vi "GetShpaeResultValue.vi"(8 "error in (no error)":errorcluster, 10 "data":variant, 11 "SetParameter":T1={"Enum_ShapeType"=enum."Circles", "MaxParticle"=1, "Descriptor"={"Set 1"=100.0, "Set 2"=10.0, "Set 3"=200.0, "Set 4"=10.0}, "Match Options"={"Rotation"=TRUE, "Scale"=FALSE, "Occlusion"=FALSE, "Range Settings"=[{"Match Constraints"=0, "Min"=0.0, "Max"=360.0}]}, "Curve Parameters"={"Extraction Mode"=0, "Edge Threshold"=75, "Edge Filter Size"=1, "Min Length"=25, "Row Search Step Size"=15, "Col Search Step Size"=15, "Max Endpoint Gap"=10, "Closed"=FALSE, "Subpixel"=FALSE}, " score"=500.0} {"score" format="%#_15g"; "Curve Parameters"."Extraction Mode" items=["Normal", "Uniform Regions"]; "Curve Parameters"."Edge Filter Size" items=["Fine", "Normal"]; "Match Options"."Range Settings"."Match Constraints" items=["Rotation Angle (degrees)", "Scale Factor (%)", "Occlusion (%)"]}) -> (0 "error out":errorcluster, 3 "ResultValues":string[](array[string]))   [LabVIEW 2019]
uses:
  Controls/ShapeDectect/Analysis_ShapeDectect_Parameter.ctl
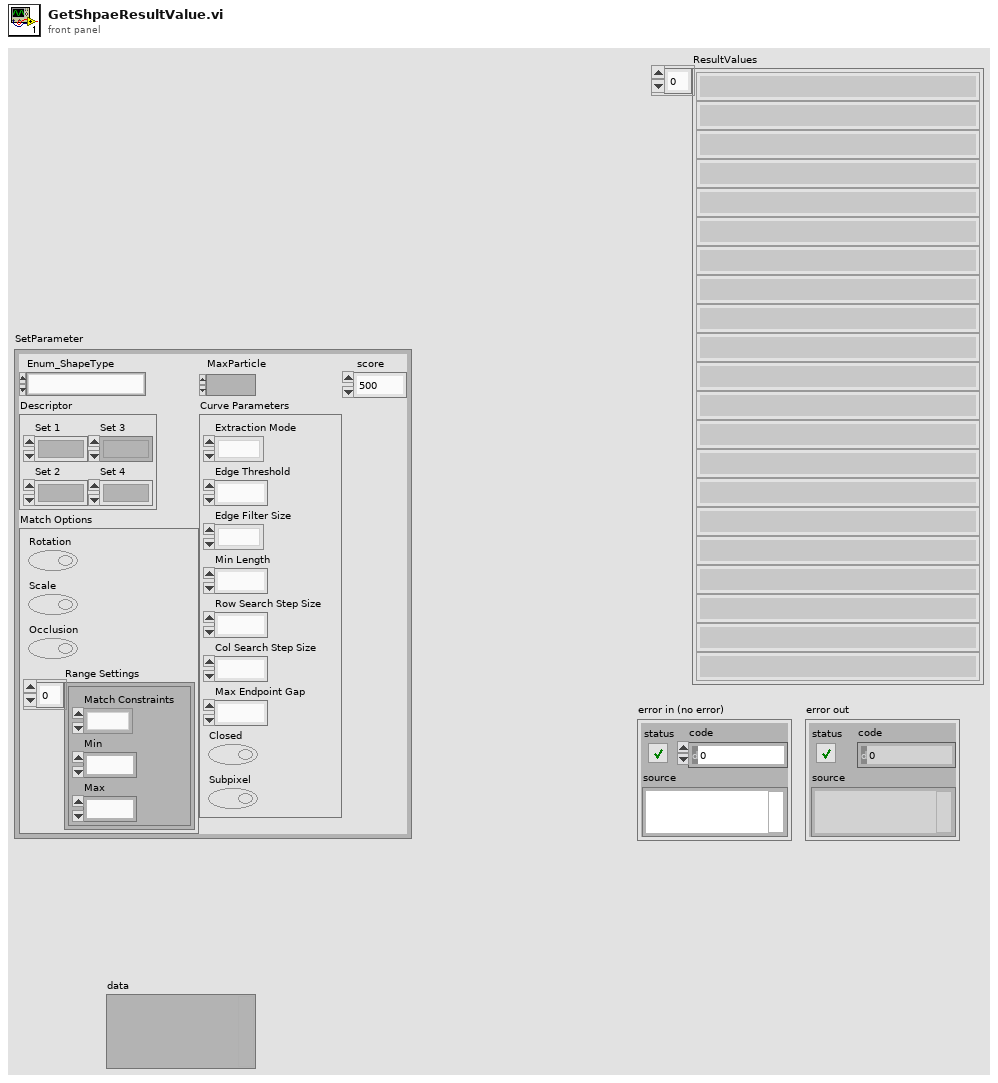
[diagram p1: front panel]
types:
  T1 = typedef "Analysis_ShapeDectect_Parameter.ctl" = cluster{"Enum_ShapeType":enum16{"Circles", "Ellipses", "Lines", "Rectangles"}, "MaxParticle":i32, "Descriptor":cluster{"Set 1":dbl, "Set 2":dbl, "Set 3":dbl, "Set 4":dbl}, "Match Options":cluster{"Rotation":bool, "Scale":bool, "Occlusion":bool, "Range Settings":cluster{"Match Constraints":u32, "Min":dbl, "Max":dbl}[]}, "Curve Parameters":cluster{"Extraction Mode":u32, "Edge Threshold":i32, "Edge Filter Size":u32, "Min Length":i32, "Row Search Step Size":i32, "Col Search Step Size":i32, "Max Endpoint Gap":i32, "Closed":bool, "Subpixel":bool}, " score":dbl}
  T2 = cluster{"Enum_ShapeType":enum16{" Circles", "Ellipses", "Lines", "Rectangles"}, "numbers":i32}
  T3 = enum16{"Circles", "Ellipses", "Lines", "Rectangles"}
  T4 = typedef "ROI Descriptor" = cluster{"Global Rectangle":i32[], "Contours":cluster{"ID":enum32{"External", "Internal"}, "Type":u32, "Coordinates":i32[]}[]}
  T5 = cluster{"Enum_ShapeType":enum16{"Circles", "Ellipses", "Lines", "Rectangles"}, "numbers":i32, "Ellipse":cluster{"ROI Descriptor out":T4, "Circle Descriptor":cluster{"Position":cluster{"X":sgl, "Y":sgl}, "Angle":dbl, "Major Radius":dbl, "Minor Radius":dbl, "Score":dbl}, "Circle Descriptor(Real)":cluster{"Position":cluster{"X":sgl, "Y":sgl}, "Orientation":dbl, "Major Radius":dbl, "Minor Radius":dbl, "Score":dbl}}[]}
  T6 = cluster{"ROI Descriptor out":T4, "Circle Descriptor":cluster{"Position":cluster{"X":sgl, "Y":sgl}, "Angle":dbl, "Major Radius":dbl, "Minor Radius":dbl, "Score":dbl}, "Circle Descriptor(Real)":cluster{"Position":cluster{"X":sgl, "Y":sgl}, "Orientation":dbl, "Major Radius":dbl, "Minor Radius":dbl, "Score":dbl}}[]
  T7 = cluster{cluster{"Global Rectangle":string[], "Contours":cluster{"ID":string, "Type":string, "Coordinates":string[]}[]}, "Circle Descriptor":cluster{"Position":cluster{"X":string, "Y":string}, "Angle":string, "Major Radius":string, "Minor Radius":string, "Score":string}, "Circle Descriptor(Real)":cluster{"Position":cluster{"X":string, "Y":string}, "Orientation":string, "Major Radius":string, "Minor Radius":string, "Score":string}}
  T8 = cluster{"Enum_ShapeType":enum16{"Circles", "Ellipses", "Lines", "Rectangles"}, "numbers":i32, "Lines":cluster{"Circle Descriptor":cluster{"Start Point":cluster{"X":sgl, "Y":sgl}, "End Point":cluster{"X":sgl, "Y":sgl}, "Length":dbl, "Angle":dbl, "Score":dbl}, "Circle Descriptor(Real)":cluster{"Start Point":cluster{"X":sgl, "Y":sgl}, "End Point":cluster{"X":sgl, "Y":sgl}, "Length":dbl, "Orientation":dbl, "Score":dbl}}[]}
  T9 = cluster{"Circle Descriptor":cluster{"Start Point":cluster{"X":sgl, "Y":sgl}, "End Point":cluster{"X":sgl, "Y":sgl}, "Length":dbl, "Angle":dbl, "Score":dbl}, "Circle Descriptor(Real)":cluster{"Start Point":cluster{"X":sgl, "Y":sgl}, "End Point":cluster{"X":sgl, "Y":sgl}, "Length":dbl, "Orientation":dbl, "Score":dbl}}[]
  T10 = cluster{"Circle Descriptor":cluster{"Start Point":cluster{"X":string, "Y":string}, "End Point":cluster{"X":string, "Y":string}, "Length":string, "Angle":string, "Score":string}, "Circle Descriptor(Real)":cluster{"Start Point":cluster{"X":string, "Y":string}, "End Point":cluster{"X":string, "Y":string}, "Length":string, "Orientation":string, "Score":string}}
  T11 = cluster{"Enum_ShapeType":enum16{"Circles", "Ellipses", "Lines", "Rectangles"}, "numbers":i32, "ReAnfle":cluster{"Rectangle Descriptor":cluster{"Corners":cluster{"X":sgl, "Y":sgl}[], "Angle":dbl, "Width":dbl, "Height":dbl, "Score":dbl}, "Rectangle Descriptor(Real)":cluster{"Corners":cluster{"X":sgl, "Y":sgl}[], "Angle":dbl, "Width":dbl, "Height":dbl, "Score":dbl}}[]}
  T12 = cluster{"Rectangle Descriptor":cluster{"Corners":cluster{"X":sgl, "Y":sgl}[], "Angle":dbl, "Width":dbl, "Height":dbl, "Score":dbl}, "Rectangle Descriptor(Real)":cluster{"Corners":cluster{"X":sgl, "Y":sgl}[], "Angle":dbl, "Width":dbl, "Height":dbl, "Score":dbl}}[]
  T13 = cluster{"Rectangle Descriptor":cluster{"Corners":cluster{"X":string, "Y":string}[], "Angle":string, "Width":string, "Height":string, "Score":string}, "Rectangle Descriptor(Real)":cluster{"Corners":cluster{"X":string, "Y":string}[], "Angle":string, "Width":string, "Height":string, "Score":string}}
  T14 = cluster{"Enum_ShapeType":enum16{"Circles", "Ellipses", "Lines", "Rectangles"}, "numbers":i32, "Circle ":cluster{"ROI Descriptor out":T4, "Circle Descriptor":cluster{"Position":cluster{"X":sgl, "Y":sgl}, "Radius":dbl, "Score":dbl}, "Circle Descriptor(Real)":cluster{"Position":cluster{"X":sgl, "Y":sgl}, "Radius":dbl, "Score":dbl}}[]}
  T15 = cluster{"ROI Descriptor out":T4, "Circle Descriptor":cluster{"Position":cluster{"X":sgl, "Y":sgl}, "Radius":dbl, "Score":dbl}, "Circle Descriptor(Real)":cluster{"Position":cluster{"X":sgl, "Y":sgl}, "Radius":dbl, "Score":dbl}}[]
  T16 = cluster{cluster{"Global Rectangle":string[], "Contours":cluster{"ID":string, "Type":string, "Coordinates":string[]}[]}, "Circle Descriptor":cluster{"Position":cluster{"X":string, "Y":string}, "Radius":string, "Score":string}, "Circle Descriptor(Real)":cluster{"Position":cluster{"X":string, "Y":string}, "Radius":string, "Score":string}}
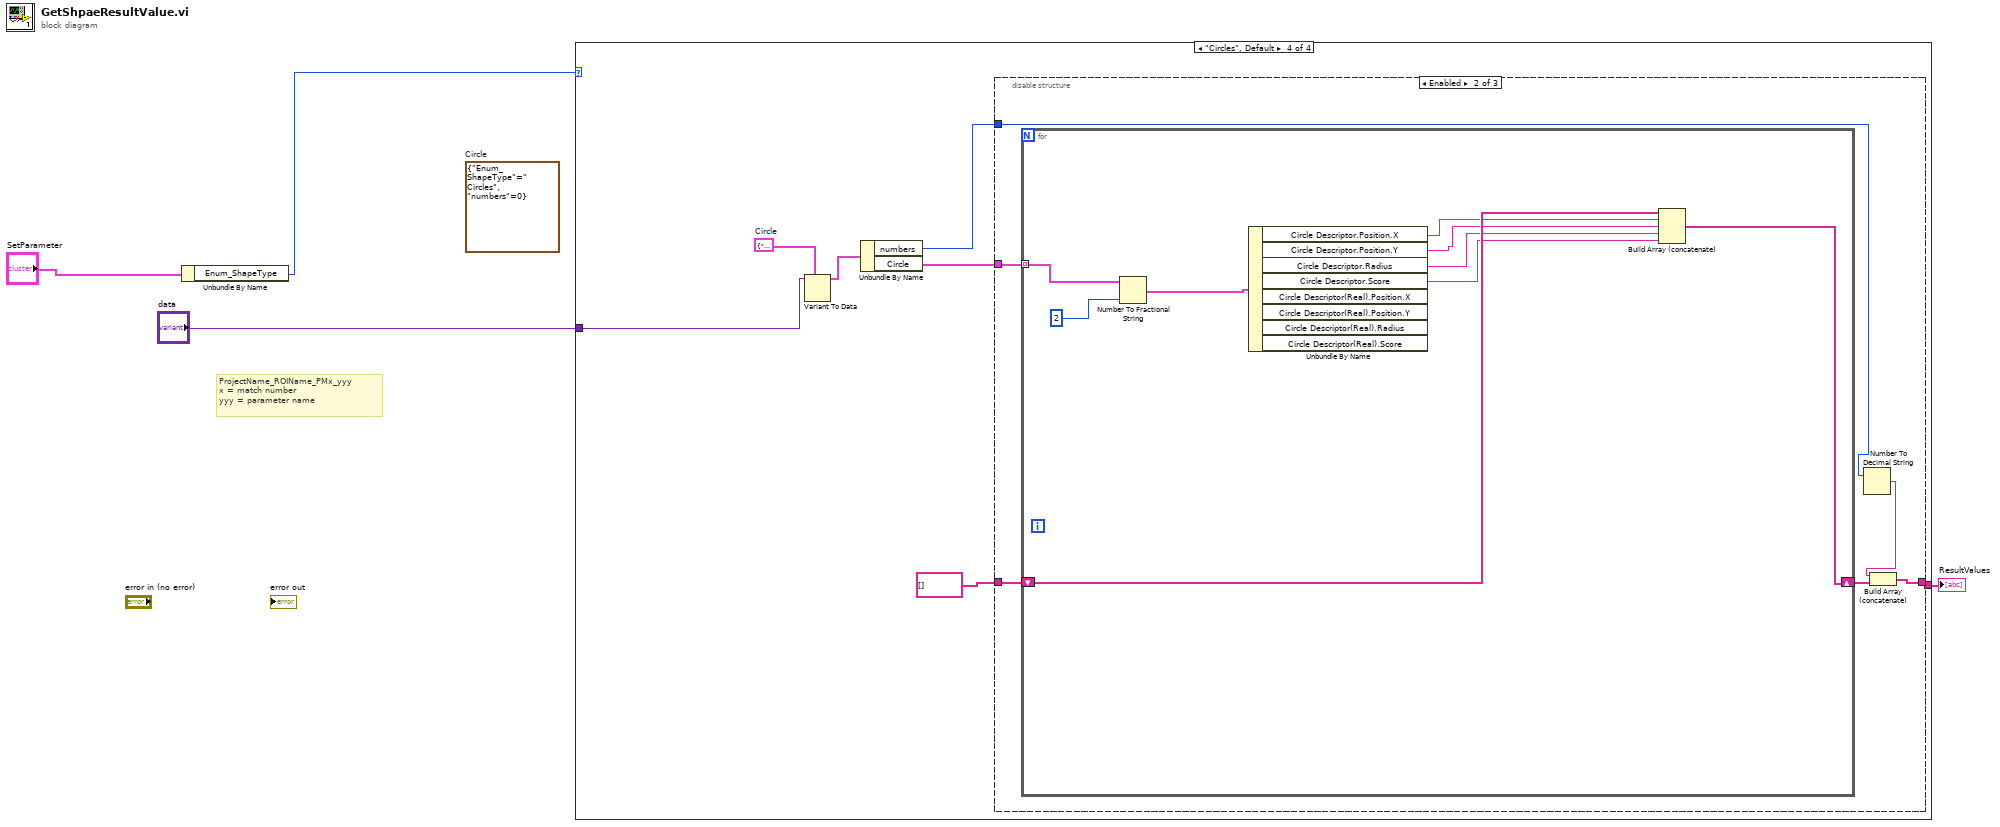
[diagram p0: block diagram]
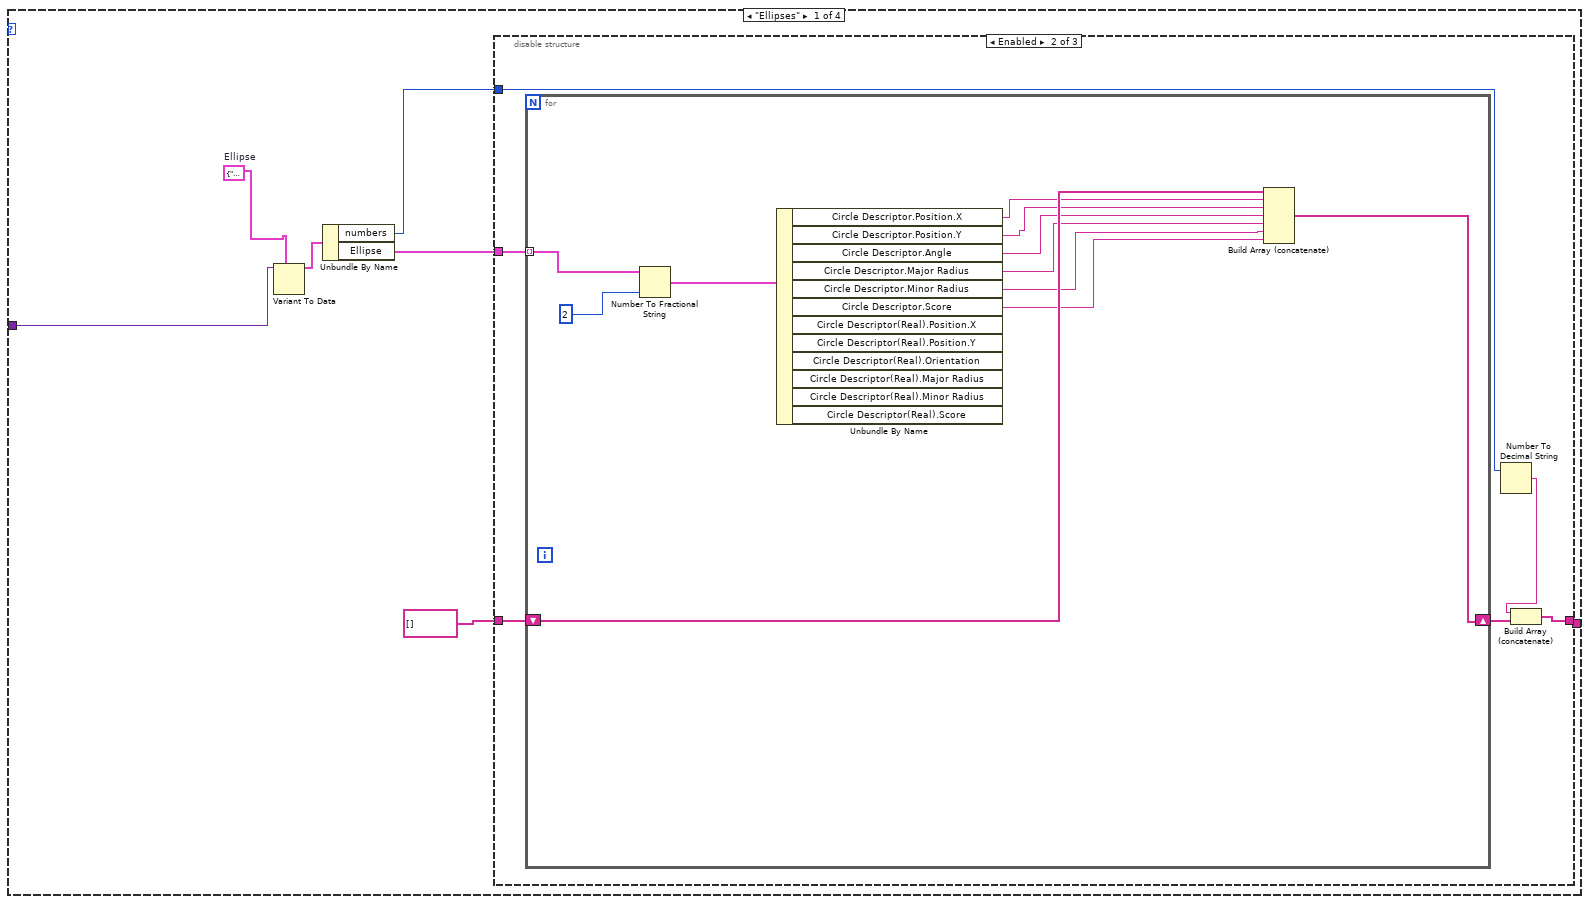
[diagram p2: hidden frame]
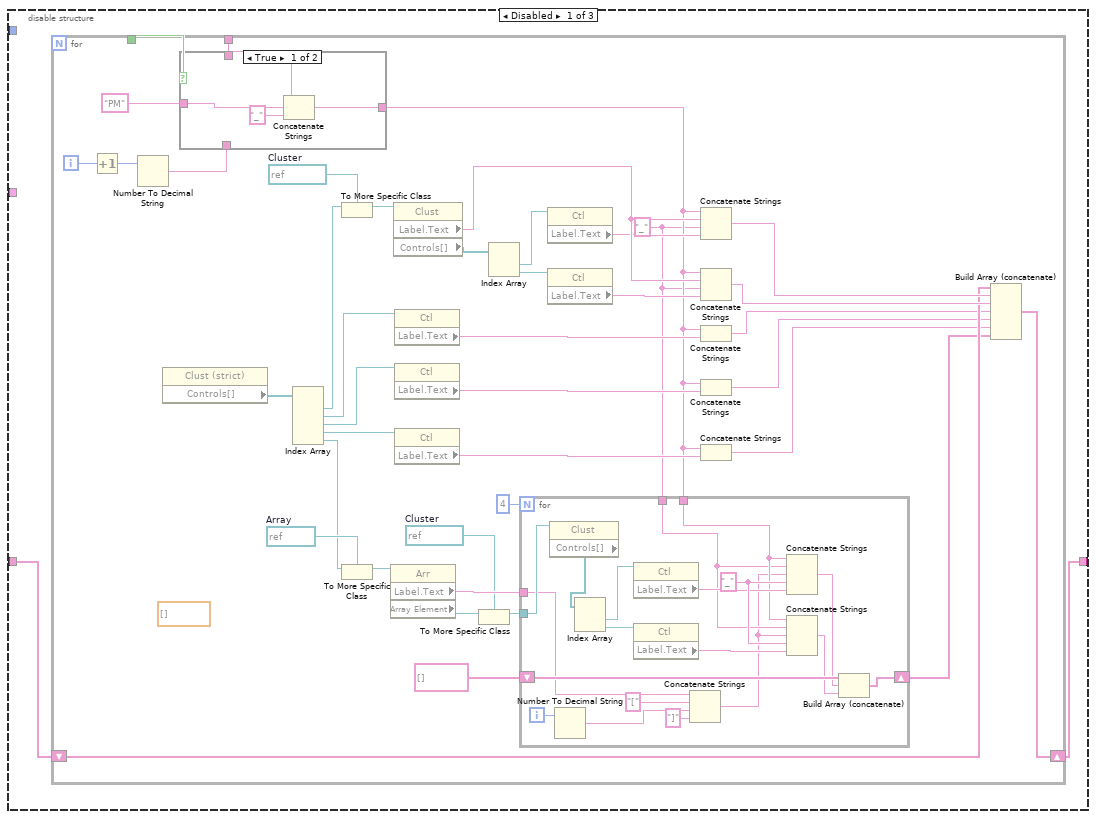
[diagram p3: hidden frame]
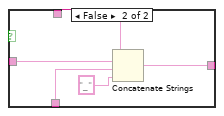
[diagram p4: hidden frame]
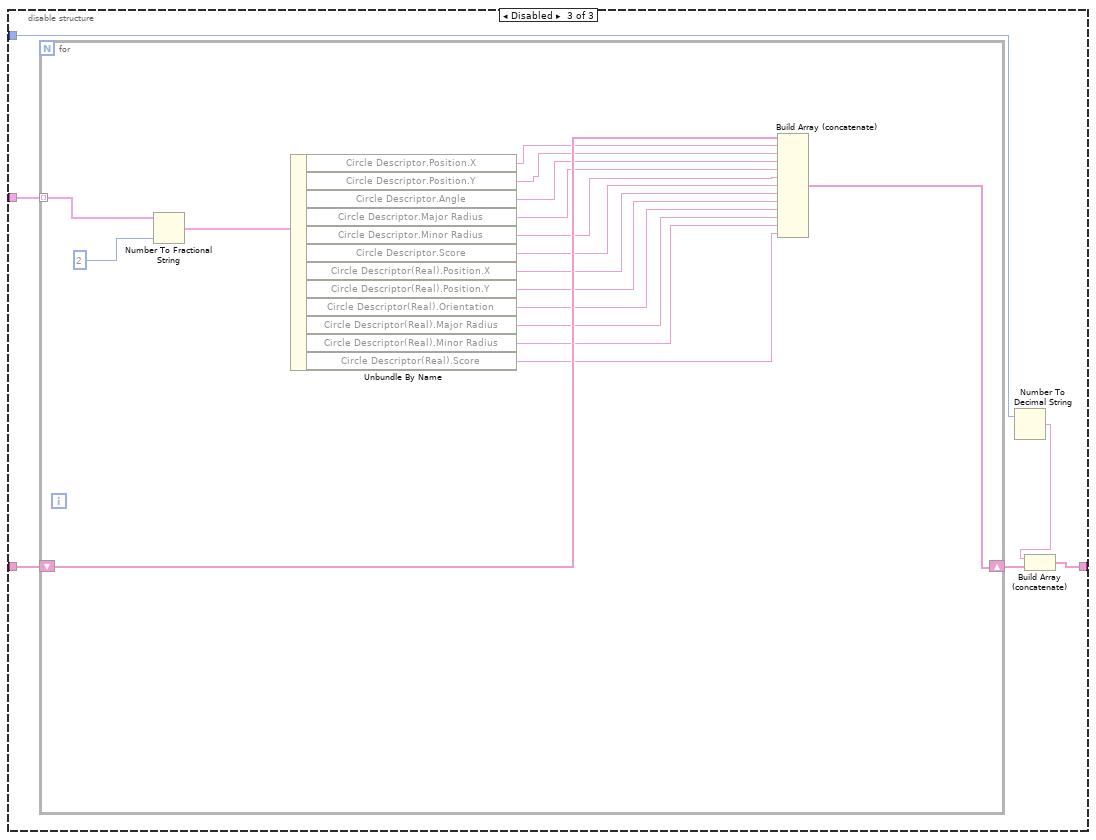
[diagram p5: hidden frame]
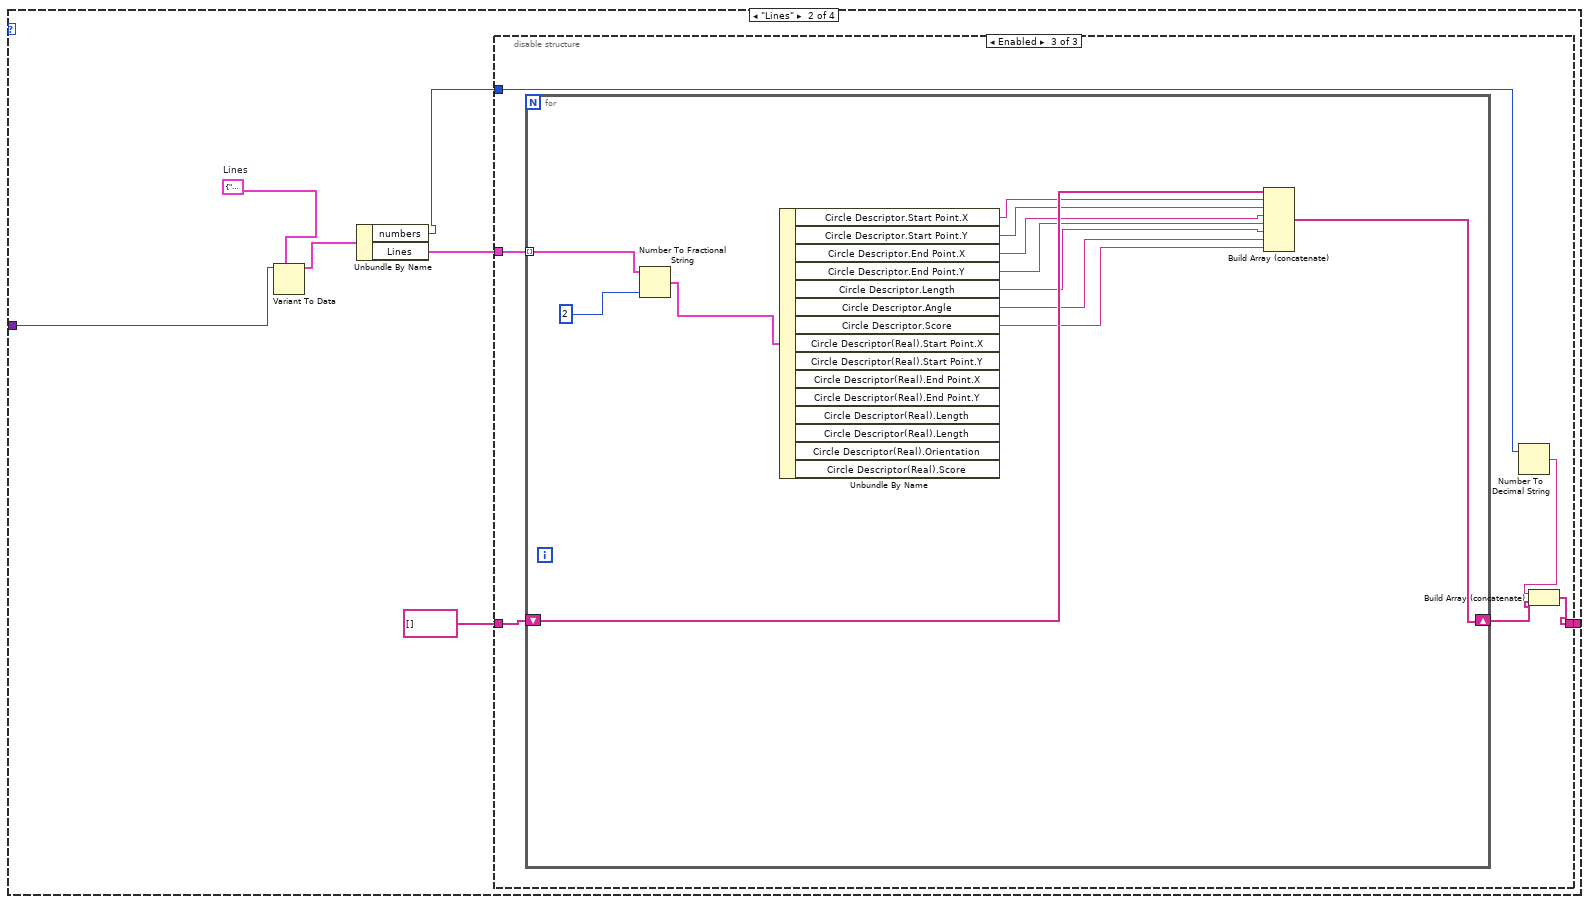
[diagram p6: hidden frame]
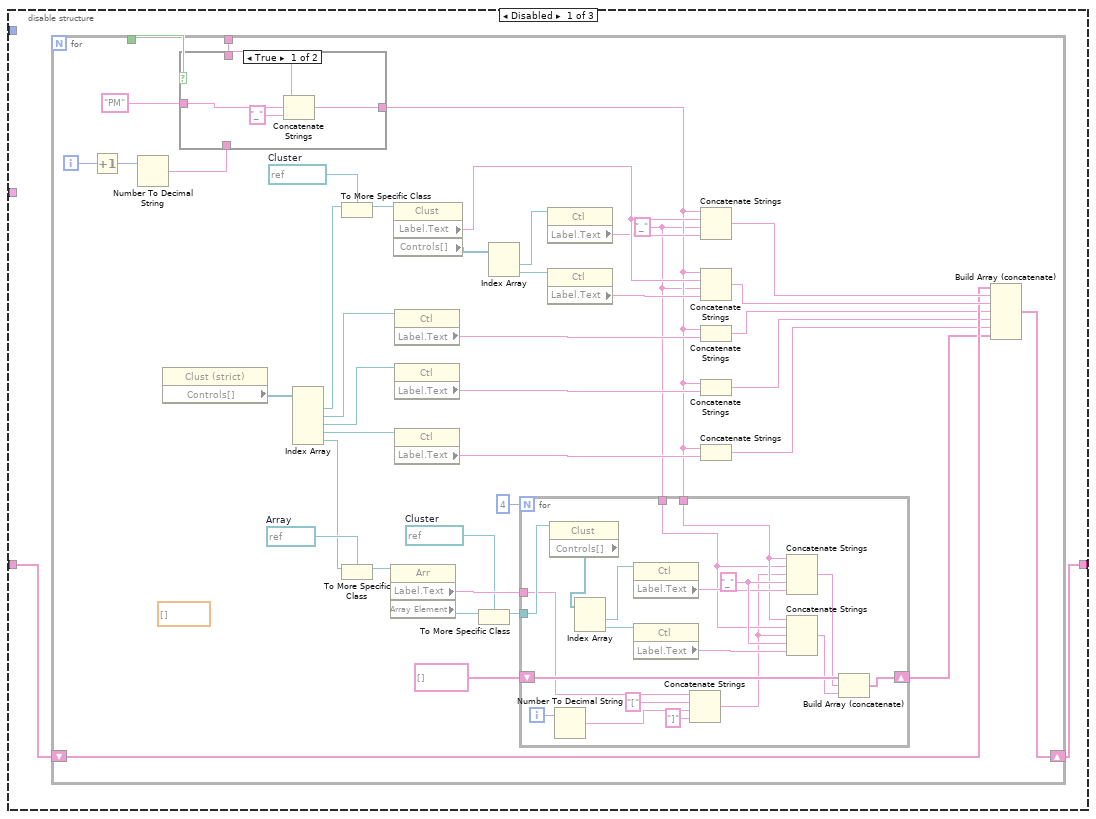
[diagram p7: hidden frame]
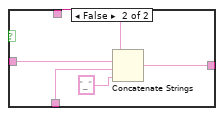
[diagram p8: hidden frame]
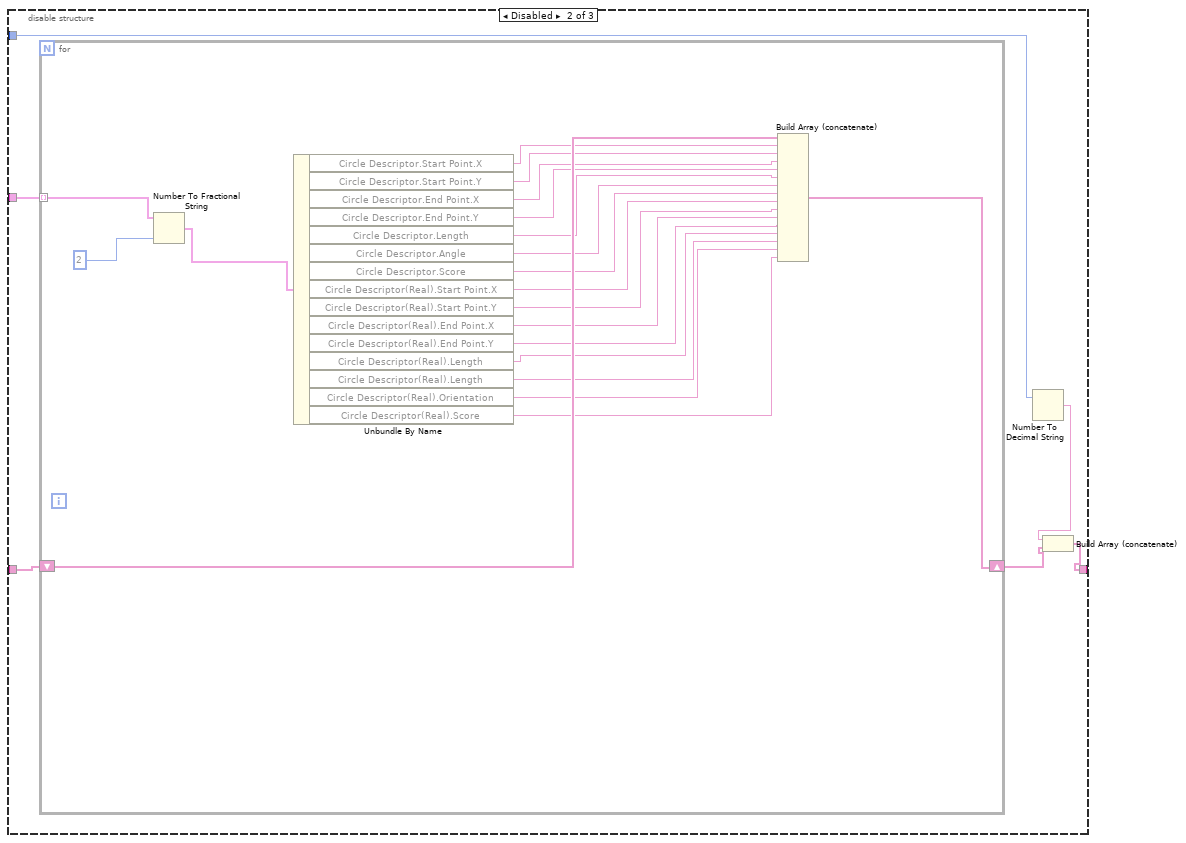
[diagram p9: hidden frame]
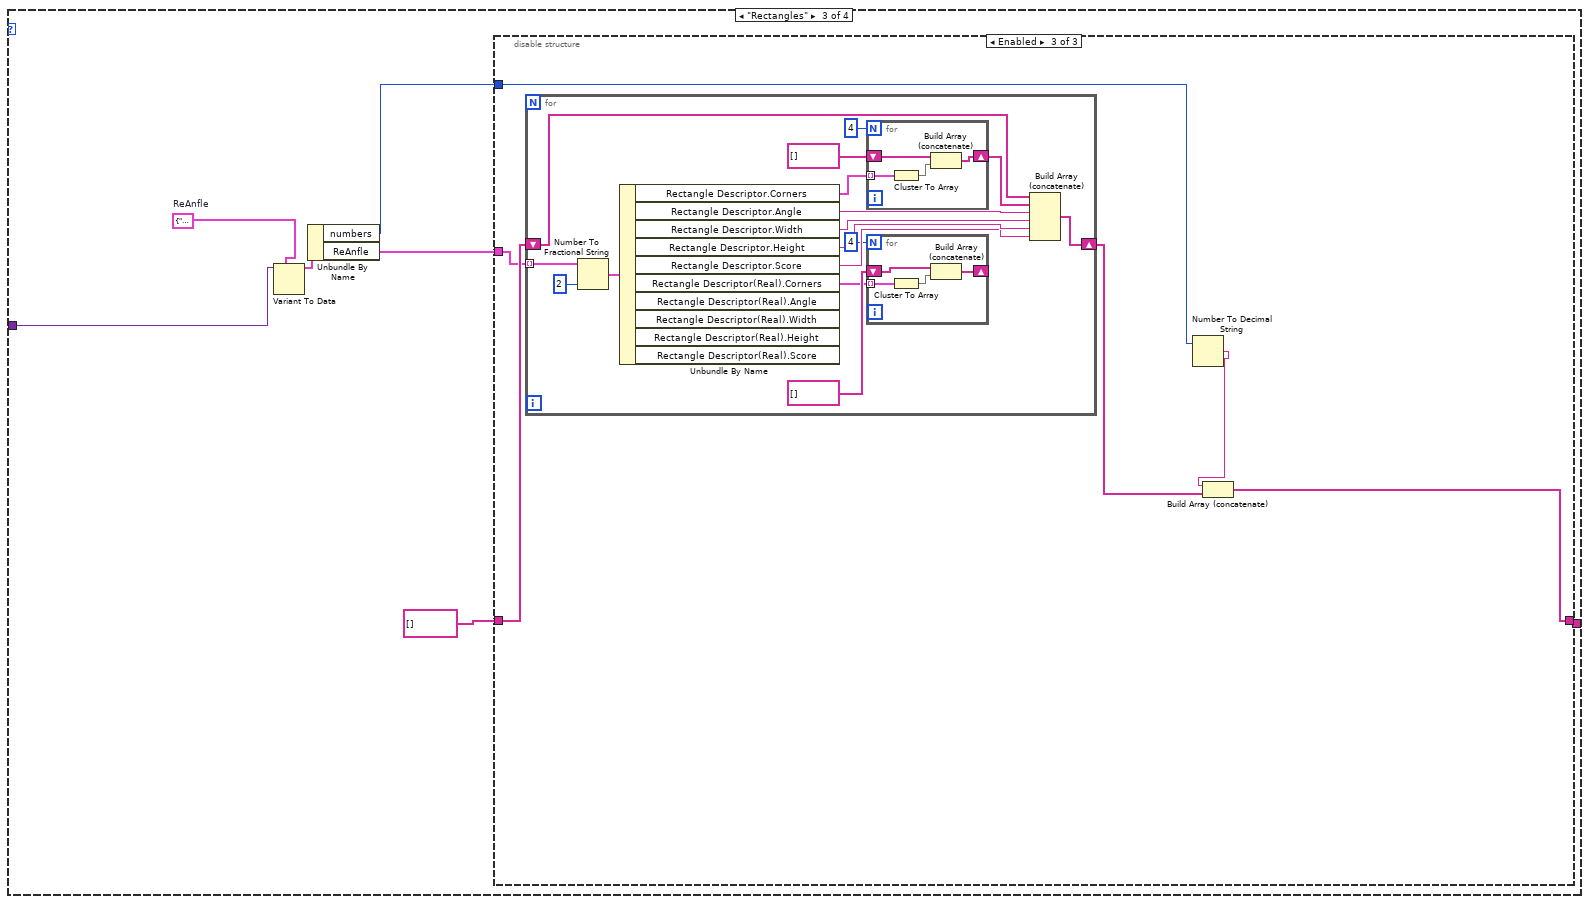
[diagram p10: hidden frame]
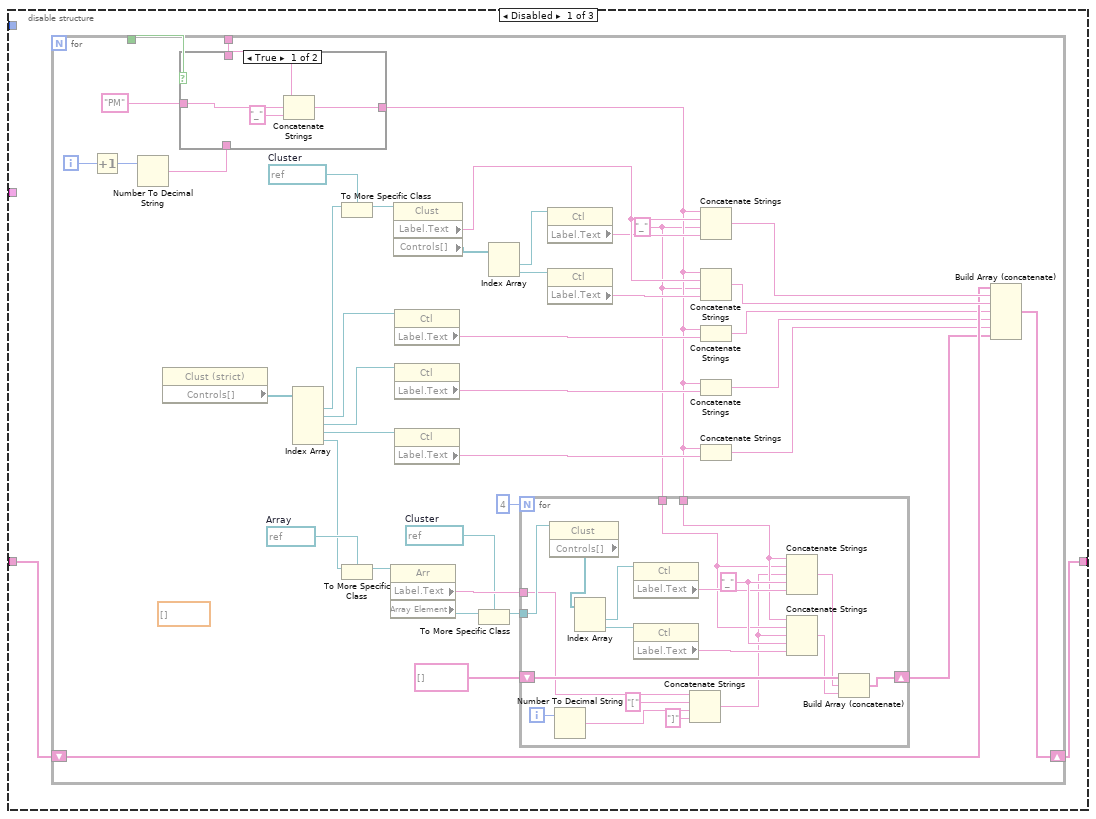
[diagram p11: hidden frame]
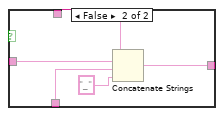
[diagram p12: hidden frame]
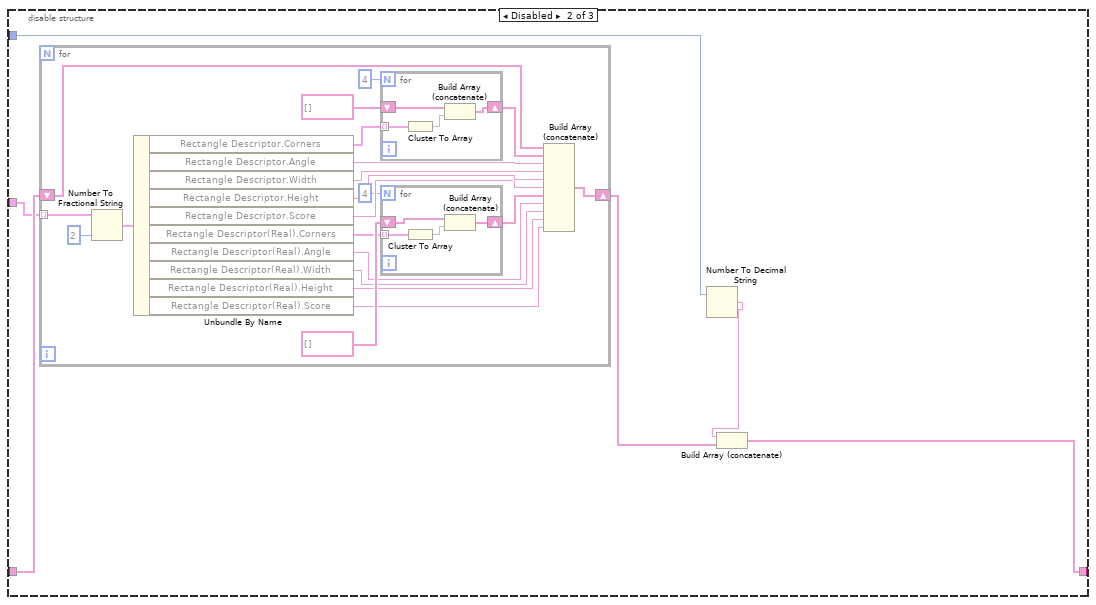
[diagram p13: hidden frame]
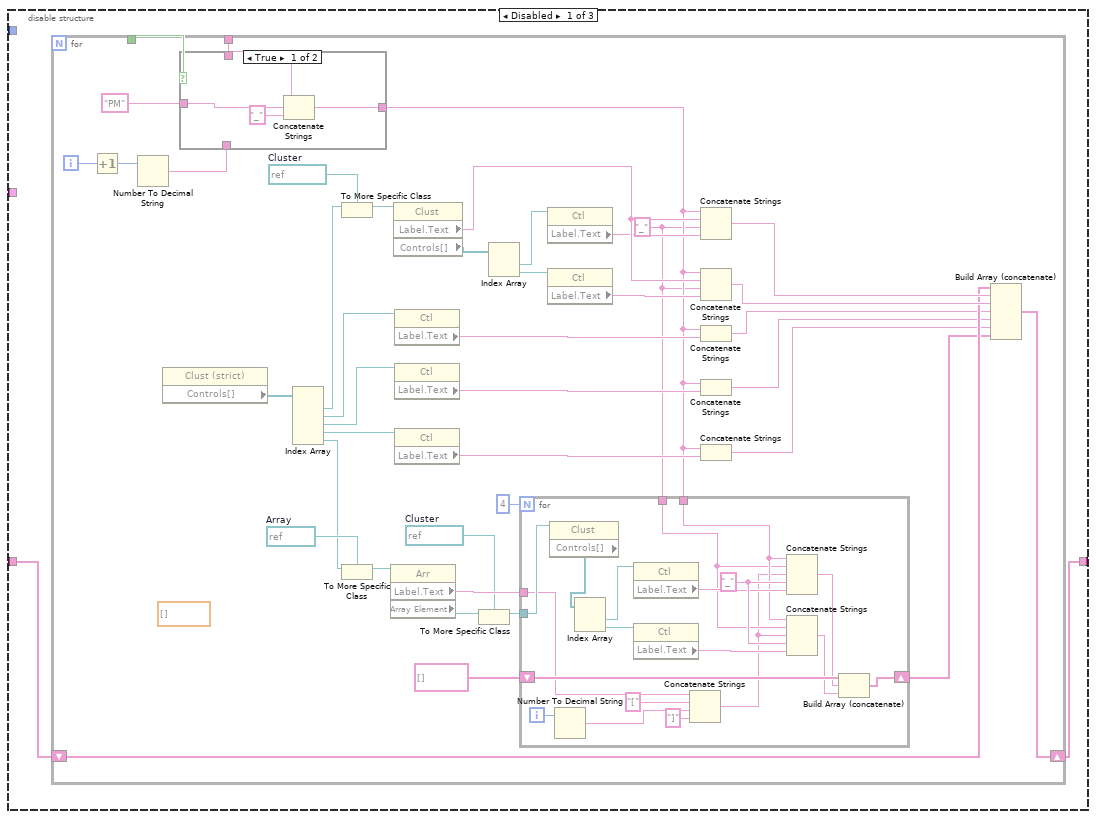
[diagram p14: hidden frame]
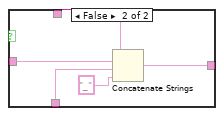
[diagram p15: hidden frame]
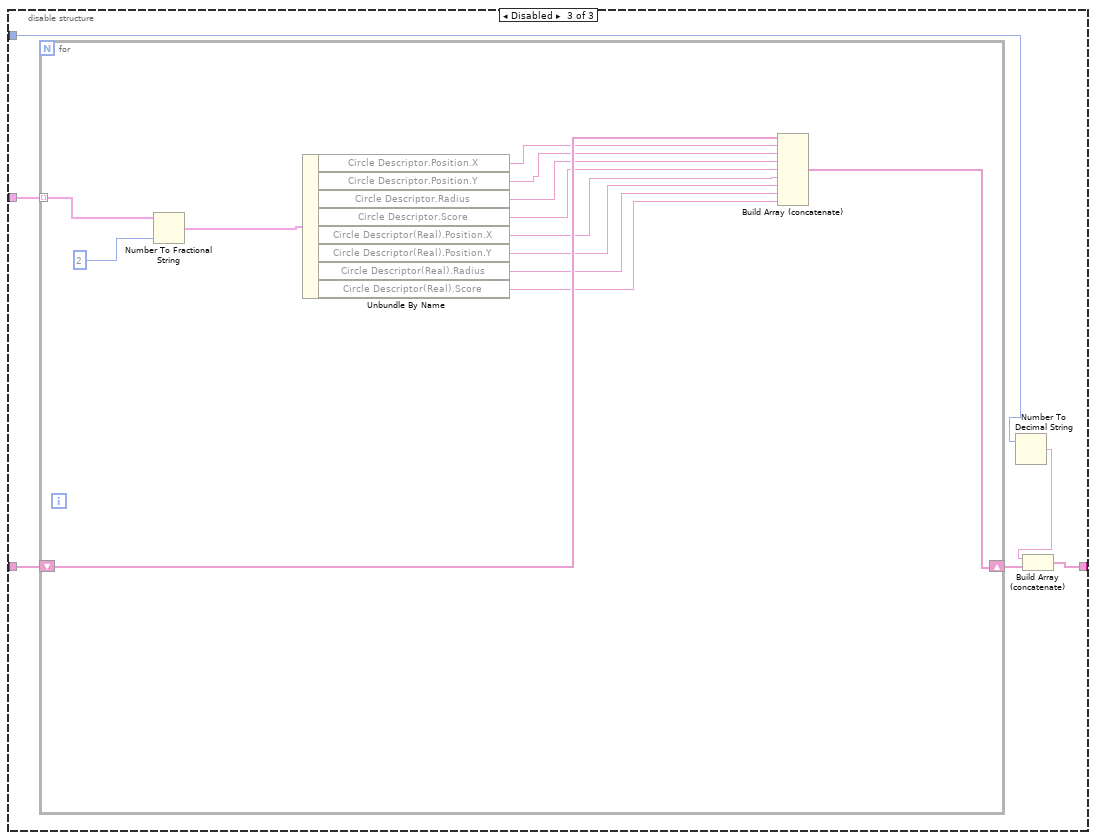
[diagram p16: hidden frame]
diagram:
  (unwired) T2 {"Enum_ShapeType"=enum." Circles", "numbers"=0}  # Circle
  # "ProjectName_ROIName_PMx_yyy\nx = match number\nyyy = parameter name"
  n1 = Unbundle By Name("SetParameter") -> ("Enum_ShapeType"=w1:T3)
  n2 = case shown="\"Circles\", Default" w1 {
    tunnel: [w10 w127 w256 w402] -> w4
    tunnel: "data" -> [w9 w131 w255 w401]
    frame "Ellipses" {
      w6 = T5 {"Enum_ShapeType"=enum."Circles", "numbers"=0, "Ellipse"=[]}  # Ellipse
      n3 = Variant To Data(type=w6, Variant=w9) -> (data=w8:T5)  [unwired: 1 in, 1 out]
      n4 = Unbundle By Name(w8) -> ("numbers"=w5:i32, "Ellipse"=w7:T6)
      n5 = disable-structure shown="Enabled" {
        disable-tunnel: string[] [] -> [w14 w91 w108]
        disable-tunnel: [w13 w87 w104] -> w10
        disable-tunnel: w7 -> [_ w89 w106]
        disable-tunnel: w5 -> [_ w88 w105]
        frame Disabled {
          n6 = for {
            N: [_] -> w15
            tunnel: _ -> [w37]
            shift-right: [w39] -> w13
            shift-left: w14 -> [w40]
            tunnel: [w38] -> w12
            i -> [w43]
            w22 = refnum<vi> refnum  # Cluster
            (unwired) dbl[] []
            w27 = refnum<vi> refnum  # Array
            w18 = "_" ("string")
            w53 = refnum<vi> refnum  # Cluster
            n7 = Increment(x=w43) -> (x+1=w42:i32)
            n8 = Number To Decimal String(number=w42) -> (decimal integer string=w36:string)  [unwired: 1 in]
            n9 = property class="Clust (strict)"() -> (reference=w57:refnum<vi>, "Controls[]"=w56:refnum<vi>[])  [unwired: 1 in, 2 out]
            n10 = case shown="True" w38 {
              tunnel: w37 -> [w80 w85]
              tunnel: w36 -> [_ w82]
              tunnel: [w79 w84] -> w19
              tunnel: "PM" ("string") -> [w78 w81]
              frame True {
                n11 = Concatenate Strings(w80, w78, "_" ("string")) -> (w79:string)
              }
              frame False {
                n12 = Concatenate Strings(w85, w81, w82, "_" ("string")) -> (w84:string)
              }
            }
            n13 = Index Array(array=w56) -> (element #1=w55:refnum<vi>, element #2=w34:refnum<vi>, element #3=w33:refnum<vi>, element #4=w46:refnum<vi>, element #5=w26:refnum<vi>)  [unwired: 5 in]
            n14 = To More Specific Class(target class=w53, reference=w55) -> (specific class reference=w54:refnum<vi>)  [unwired: 1 in, 1 out]
            n15 = To More Specific Class(target class=w27, reference=w26) -> (specific class reference=w25:refnum<vi>)  [unwired: 1 in, 1 out]
            n16 = property class="Arr"(reference=w25) -> ("Label.Text"=w24:string, "Array Element"=w21:refnum<vi>)  [unwired: 1 in, 2 out]
            n17 = property class="Clust"(reference=w54) -> ("Label.Text"=w49:string, "Controls[]"=w52:refnum<vi>[])  [unwired: 1 in, 2 out]
            n18 = property class="Ctl"(reference=w34) -> ("Label.Text"=w32:string)  [unwired: 1 in, 2 out]
            n19 = property class="Ctl"(reference=w33) -> ("Label.Text"=w31:string)  [unwired: 1 in, 2 out]
            n20 = property class="Ctl"(reference=w46) -> ("Label.Text"=w41:string)  [unwired: 1 in, 2 out]
            n21 = To More Specific Class(target class=w22, reference=w21) -> (specific class reference=w20:refnum<vi>)  [unwired: 1 in, 1 out]
            n22 = Index Array(array=w52) -> (element #1=w51:refnum<vi>, element #2=w50:refnum<vi>)  [unwired: 2 in]
            n23 = for {
              N: 4 -> [_]
              tunnel: w24 -> [w62]
              tunnel: w20 -> [w76]
              tunnel: w19 -> [w69]
              tunnel: w18 -> [w68]
              shift-right: [w64] -> w16
              shift-left: string[] [] -> [w67]
              i -> [w63]
              w75 = "_" ("string")
              n24 = property class="Clust"(reference=w76) -> ("Controls[]"=w70:refnum<vi>[])  [unwired: 1 in, 2 out]
              n25 = Number To Decimal String(number=w63) -> (decimal integer string=w60:string)  [unwired: 1 in]
              n26 = Index Array(array=w70) -> (element #1=w71:refnum<vi>, element #2=w72:refnum<vi>)  [unwired: 2 in]
              n27 = property class="Ctl"(reference=w71) -> ("Label.Text"=w73:string)  [unwired: 1 in, 2 out]
              n28 = property class="Ctl"(reference=w72) -> ("Label.Text"=w74:string)  [unwired: 1 in, 2 out]
              n29 = Concatenate Strings(w62, "[" ("string"), w60, "]" ("string")) -> (w58:string)
              n30 = Concatenate Strings(w69, w68, w58, w75, w73) -> (w66:string)
              n31 = Concatenate Strings(w69, w68, w58, w75, w74) -> (w65:string)
              n32 = Build Array (concatenate)(w67, w66, w65) -> (w64:string[])
            }
            n33 = property class="Ctl"(reference=w51) -> ("Label.Text"=w48:string)  [unwired: 1 in, 2 out]
            n34 = property class="Ctl"(reference=w50) -> ("Label.Text"=w47:string)  [unwired: 1 in, 2 out]
            n35 = Concatenate Strings(w19, w49, w18, w48) -> (w45:string)
            n36 = Concatenate Strings(w19, w49, w18, w47) -> (w44:string)
            n37 = Concatenate Strings(w19, w32) -> (w28:string)
            n38 = Concatenate Strings(w19, w31) -> (w29:string)
            n39 = Concatenate Strings(w19, w41) -> (w30:string)
            n40 = Build Array (concatenate)(w40, w45, w44, w28, w29, w30, w16) -> (w39:string[])
          }
        }
        frame Enabled {
          n41 = for {
            shift-right: [w92] -> w90
            shift-left: w91 -> [w102]
            tunnel: w89 -> [w100] mode=indexing
            n42 = Number To Fractional String(number=w100, precision (6)=2) -> (F-format string=w99:T7)  [unwired: 2 in]
            n43 = Unbundle By Name(w99) -> ("Circle Descriptor.Position.X"=w98:string, "Circle Descriptor.Position.Y"=w97:string, "Circle Descriptor.Angle"=w96:string, "Circle Descriptor.Major Radius"=w95:string, "Circle Descriptor.Minor Radius"=w94:string, "Circle Descriptor.Score"=w93:string)  [unwired: 6 out]
            n44 = Build Array (concatenate)(w102, w98, w97, w96, w95, w94, w93) -> (w92:string[])
          }
          n45 = Number To Decimal String(number=w88) -> (decimal integer string=w86:string)  [unwired: 1 in]
          n46 = Build Array (concatenate)(w86, w90) -> (w87:string[])
        }
        frame Disabled {
          n47 = for {
            shift-right: [w109] -> w107
            shift-left: w108 -> [w125]
            tunnel: w106 -> [w123] mode=indexing
            n48 = Number To Fractional String(number=w123, precision (6)=2) -> (F-format string=w122:T7)  [unwired: 2 in]
            n49 = Unbundle By Name(w122) -> ("Circle Descriptor.Position.X"=w121:string, "Circle Descriptor.Position.Y"=w120:string, "Circle Descriptor.Angle"=w119:string, "Circle Descriptor.Major Radius"=w118:string, "Circle Descriptor.Minor Radius"=w117:string, "Circle Descriptor.Score"=w116:string, "Circle Descriptor(Real).Position.X"=w115:string, "Circle Descriptor(Real).Position.Y"=w114:string, "Circle Descriptor(Real).Orientation"=w113:string, "Circle Descriptor(Real).Major Radius"=w112:string, "Circle Descriptor(Real).Minor Radius"=w111:string, "Circle Descriptor(Real).Score"=w110:string)
            n50 = Build Array (concatenate)(w125, w121, w120, w119, w118, w117, w116, w115, w114, w113, w112, w111, w110) -> (w109:string[])
          }
          n51 = Number To Decimal String(number=w105) -> (decimal integer string=w103:string)  [unwired: 1 in]
          n52 = Build Array (concatenate)(w103, w107) -> (w104:string[])
        }
      }
    }
    frame "Lines" {
      w128 = T8 {"Enum_ShapeType"=enum."Circles", "numbers"=0, "Lines"=[]}  # Lines
      n53 = Variant To Data(type=w128, Variant=w131) -> (data=w130:T8)  [unwired: 1 in, 1 out]
      n54 = Unbundle By Name(w130) -> ("numbers"=w126:i32, "Lines"=w129:T9)
      n55 = disable-structure shown="Enabled" {
        disable-tunnel: string[] [] -> [w135 w212 w238]
        disable-tunnel: w129 -> [_ w211 w237]
        disable-tunnel: [w134 w209 w235] -> w127
        disable-tunnel: w126 -> [_ w207 w233]
        frame Disabled {
          n56 = for {
            N: [_] -> w136
            tunnel: _ -> [w158]
            shift-right: [w160] -> w134
            shift-left: w135 -> [w161]
            tunnel: [w159] -> w133
            i -> [w164]
            w143 = refnum<vi> refnum  # Cluster
            (unwired) dbl[] []
            w148 = refnum<vi> refnum  # Array
            w139 = "_" ("string")
            w174 = refnum<vi> refnum  # Cluster
            n57 = Increment(x=w164) -> (x+1=w163:i32)
            n58 = Number To Decimal String(number=w163) -> (decimal integer string=w157:string)  [unwired: 1 in]
            n59 = property class="Clust (strict)"() -> (reference=w178:refnum<vi>, "Controls[]"=w177:refnum<vi>[])  [unwired: 1 in, 2 out]
            n60 = case shown="True" w159 {
              tunnel: w158 -> [w201 w206]
              tunnel: w157 -> [_ w203]
              tunnel: [w200 w205] -> w140
              tunnel: "PM" ("string") -> [w199 w202]
              frame True {
                n61 = Concatenate Strings(w201, w199, "_" ("string")) -> (w200:string)
              }
              frame False {
                n62 = Concatenate Strings(w206, w202, w203, "_" ("string")) -> (w205:string)
              }
            }
            n63 = Index Array(array=w177) -> (element #1=w176:refnum<vi>, element #2=w155:refnum<vi>, element #3=w154:refnum<vi>, element #4=w167:refnum<vi>, element #5=w147:refnum<vi>)  [unwired: 5 in]
            n64 = To More Specific Class(target class=w174, reference=w176) -> (specific class reference=w175:refnum<vi>)  [unwired: 1 in, 1 out]
            n65 = To More Specific Class(target class=w148, reference=w147) -> (specific class reference=w146:refnum<vi>)  [unwired: 1 in, 1 out]
            n66 = property class="Arr"(reference=w146) -> ("Label.Text"=w145:string, "Array Element"=w142:refnum<vi>)  [unwired: 1 in, 2 out]
            n67 = property class="Clust"(reference=w175) -> ("Label.Text"=w170:string, "Controls[]"=w173:refnum<vi>[])  [unwired: 1 in, 2 out]
            n68 = property class="Ctl"(reference=w155) -> ("Label.Text"=w153:string)  [unwired: 1 in, 2 out]
            n69 = property class="Ctl"(reference=w154) -> ("Label.Text"=w152:string)  [unwired: 1 in, 2 out]
            n70 = property class="Ctl"(reference=w167) -> ("Label.Text"=w162:string)  [unwired: 1 in, 2 out]
            n71 = To More Specific Class(target class=w143, reference=w142) -> (specific class reference=w141:refnum<vi>)  [unwired: 1 in, 1 out]
            n72 = Index Array(array=w173) -> (element #1=w172:refnum<vi>, element #2=w171:refnum<vi>)  [unwired: 2 in]
            n73 = for {
              N: 4 -> [_]
              tunnel: w145 -> [w183]
              tunnel: w141 -> [w197]
              tunnel: w140 -> [w190]
              tunnel: w139 -> [w189]
              shift-right: [w185] -> w137
              shift-left: string[] [] -> [w188]
              i -> [w184]
              w196 = "_" ("string")
              n74 = property class="Clust"(reference=w197) -> ("Controls[]"=w191:refnum<vi>[])  [unwired: 1 in, 2 out]
              n75 = Number To Decimal String(number=w184) -> (decimal integer string=w181:string)  [unwired: 1 in]
              n76 = Index Array(array=w191) -> (element #1=w192:refnum<vi>, element #2=w193:refnum<vi>)  [unwired: 2 in]
              n77 = property class="Ctl"(reference=w192) -> ("Label.Text"=w194:string)  [unwired: 1 in, 2 out]
              n78 = property class="Ctl"(reference=w193) -> ("Label.Text"=w195:string)  [unwired: 1 in, 2 out]
              n79 = Concatenate Strings(w183, "[" ("string"), w181, "]" ("string")) -> (w179:string)
              n80 = Concatenate Strings(w190, w189, w179, w196, w194) -> (w187:string)
              n81 = Concatenate Strings(w190, w189, w179, w196, w195) -> (w186:string)
              n82 = Build Array (concatenate)(w188, w187, w186) -> (w185:string[])
            }
            n83 = property class="Ctl"(reference=w172) -> ("Label.Text"=w169:string)  [unwired: 1 in, 2 out]
            n84 = property class="Ctl"(reference=w171) -> ("Label.Text"=w168:string)  [unwired: 1 in, 2 out]
            n85 = Concatenate Strings(w140, w170, w139, w169) -> (w166:string)
            n86 = Concatenate Strings(w140, w170, w139, w168) -> (w165:string)
            n87 = Concatenate Strings(w140, w153) -> (w149:string)
            n88 = Concatenate Strings(w140, w152) -> (w150:string)
            n89 = Concatenate Strings(w140, w162) -> (w151:string)
            n90 = Build Array (concatenate)(w161, w166, w165, w149, w150, w151, w137) -> (w160:string[])
          }
        }
        frame Disabled {
          n91 = for {
            shift-right: [w230] -> w210
            shift-left: w212 -> [w232]
            tunnel: w211 -> [w229] mode=indexing
            n92 = Number To Fractional String(number=w229, precision (6)=2) -> (F-format string=w228:T10)  [unwired: 2 in]
            n93 = Unbundle By Name(w228) -> ("Circle Descriptor.Start Point.X"=w227:string, "Circle Descriptor.Start Point.Y"=w226:string, "Circle Descriptor.End Point.X"=w225:string, "Circle Descriptor.End Point.Y"=w224:string, "Circle Descriptor.Length"=w223:string, "Circle Descriptor.Angle"=w222:string, "Circle Descriptor.Score"=w221:string, "Circle Descriptor(Real).Start Point.X"=w220:string, "Circle Descriptor(Real).Start Point.Y"=w219:string, "Circle Descriptor(Real).End Point.X"=w218:string, "Circle Descriptor(Real).End Point.Y"=w217:string, "Circle Descriptor(Real).Length"=w216:string, "Circle Descriptor(Real).Length"=w215:string, "Circle Descriptor(Real).Orientation"=w214:string, "Circle Descriptor(Real).Score"=w213:string)
            n94 = Build Array (concatenate)(w232, w227, w226, w225, w224, w223, w222, w221, w220, w219, w218, w217, w216, w215, w214, w213) -> (w230:string[])
          }
          n95 = Number To Decimal String(number=w207) -> (decimal integer string=w208:string)  [unwired: 1 in]
          n96 = Build Array (concatenate)(w208, w210) -> (w209:string[])
        }
        frame Enabled {
          n97 = for {
            shift-right: [w248] -> w236
            shift-left: w238 -> [w250]
            tunnel: w237 -> [w247] mode=indexing
            n98 = Number To Fractional String(number=w247, precision (6)=2) -> (F-format string=w246:T10)  [unwired: 2 in]
            n99 = Unbundle By Name(w246) -> ("Circle Descriptor.Start Point.X"=w245:string, "Circle Descriptor.Start Point.Y"=w244:string, "Circle Descriptor.End Point.X"=w243:string, "Circle Descriptor.End Point.Y"=w242:string, "Circle Descriptor.Length"=w241:string, "Circle Descriptor.Angle"=w240:string, "Circle Descriptor.Score"=w239:string)  [unwired: 8 out]
            n100 = Build Array (concatenate)(w250, w245, w244, w243, w242, w241, w240, w239) -> (w248:string[])
          }
          n101 = Number To Decimal String(number=w233) -> (decimal integer string=w234:string)  [unwired: 1 in]
          n102 = Build Array (concatenate)(w234, w236) -> (w235:string[])
        }
      }
    }
    frame "Rectangles" {
      w253 = T11 {"Enum_ShapeType"=enum."Circles", "numbers"=0, "ReAnfle"=[]}  # ReAnfle
      n103 = Variant To Data(type=w253, Variant=w255) -> (data=w254:T11)  [unwired: 1 in, 1 out]
      n104 = Unbundle By Name(w254) -> ("numbers"=w252:i32, "ReAnfle"=w251:T12)
      n105 = disable-structure shown="Enabled" {
        disable-tunnel: string[] [] -> [w260 w337 w372]
        disable-tunnel: [w259 w332 w367] -> w256
        disable-tunnel: w251 -> [_ w336 w371]
        disable-tunnel: w252 -> [_ w333 w368]
        frame Disabled {
          n106 = for {
            N: [_] -> w261
            tunnel: _ -> [w283]
            shift-right: [w285] -> w259
            shift-left: w260 -> [w286]
            tunnel: [w284] -> w258
            i -> [w289]
            w268 = refnum<vi> refnum  # Cluster
            (unwired) dbl[] []
            w273 = refnum<vi> refnum  # Array
            w264 = "_" ("string")
            w299 = refnum<vi> refnum  # Cluster
            n107 = Increment(x=w289) -> (x+1=w288:i32)
            n108 = Number To Decimal String(number=w288) -> (decimal integer string=w282:string)  [unwired: 1 in]
            n109 = property class="Clust (strict)"() -> (reference=w303:refnum<vi>, "Controls[]"=w302:refnum<vi>[])  [unwired: 1 in, 2 out]
            n110 = case shown="True" w284 {
              tunnel: w283 -> [w326 w331]
              tunnel: w282 -> [_ w328]
              tunnel: [w325 w330] -> w265
              tunnel: "PM" ("string") -> [w324 w327]
              frame True {
                n111 = Concatenate Strings(w326, w324, "_" ("string")) -> (w325:string)
              }
              frame False {
                n112 = Concatenate Strings(w331, w327, w328, "_" ("string")) -> (w330:string)
              }
            }
            n113 = Index Array(array=w302) -> (element #1=w301:refnum<vi>, element #2=w280:refnum<vi>, element #3=w279:refnum<vi>, element #4=w292:refnum<vi>, element #5=w272:refnum<vi>)  [unwired: 5 in]
            n114 = To More Specific Class(target class=w299, reference=w301) -> (specific class reference=w300:refnum<vi>)  [unwired: 1 in, 1 out]
            n115 = To More Specific Class(target class=w273, reference=w272) -> (specific class reference=w271:refnum<vi>)  [unwired: 1 in, 1 out]
            n116 = property class="Arr"(reference=w271) -> ("Label.Text"=w270:string, "Array Element"=w267:refnum<vi>)  [unwired: 1 in, 2 out]
            n117 = property class="Clust"(reference=w300) -> ("Label.Text"=w295:string, "Controls[]"=w298:refnum<vi>[])  [unwired: 1 in, 2 out]
            n118 = property class="Ctl"(reference=w280) -> ("Label.Text"=w278:string)  [unwired: 1 in, 2 out]
            n119 = property class="Ctl"(reference=w279) -> ("Label.Text"=w277:string)  [unwired: 1 in, 2 out]
            n120 = property class="Ctl"(reference=w292) -> ("Label.Text"=w287:string)  [unwired: 1 in, 2 out]
            n121 = To More Specific Class(target class=w268, reference=w267) -> (specific class reference=w266:refnum<vi>)  [unwired: 1 in, 1 out]
            n122 = Index Array(array=w298) -> (element #1=w297:refnum<vi>, element #2=w296:refnum<vi>)  [unwired: 2 in]
            n123 = for {
              N: 4 -> [_]
              tunnel: w270 -> [w308]
              tunnel: w266 -> [w322]
              tunnel: w265 -> [w315]
              tunnel: w264 -> [w314]
              shift-right: [w310] -> w262
              shift-left: string[] [] -> [w313]
              i -> [w309]
              w321 = "_" ("string")
              n124 = property class="Clust"(reference=w322) -> ("Controls[]"=w316:refnum<vi>[])  [unwired: 1 in, 2 out]
              n125 = Number To Decimal String(number=w309) -> (decimal integer string=w306:string)  [unwired: 1 in]
              n126 = Index Array(array=w316) -> (element #1=w317:refnum<vi>, element #2=w318:refnum<vi>)  [unwired: 2 in]
              n127 = property class="Ctl"(reference=w317) -> ("Label.Text"=w319:string)  [unwired: 1 in, 2 out]
              n128 = property class="Ctl"(reference=w318) -> ("Label.Text"=w320:string)  [unwired: 1 in, 2 out]
              n129 = Concatenate Strings(w308, "[" ("string"), w306, "]" ("string")) -> (w304:string)
              n130 = Concatenate Strings(w315, w314, w304, w321, w319) -> (w312:string)
              n131 = Concatenate Strings(w315, w314, w304, w321, w320) -> (w311:string)
              n132 = Build Array (concatenate)(w313, w312, w311) -> (w310:string[])
            }
            n133 = property class="Ctl"(reference=w297) -> ("Label.Text"=w294:string)  [unwired: 1 in, 2 out]
            n134 = property class="Ctl"(reference=w296) -> ("Label.Text"=w293:string)  [unwired: 1 in, 2 out]
            n135 = Concatenate Strings(w265, w295, w264, w294) -> (w291:string)
            n136 = Concatenate Strings(w265, w295, w264, w293) -> (w290:string)
            n137 = Concatenate Strings(w265, w278) -> (w274:string)
            n138 = Concatenate Strings(w265, w277) -> (w275:string)
            n139 = Concatenate Strings(w265, w287) -> (w276:string)
            n140 = Build Array (concatenate)(w286, w291, w290, w274, w275, w276, w262) -> (w285:string[])
          }
        }
        frame Disabled {
          n141 = for {
            shift-right: [w356] -> w335
            shift-left: w337 -> [w358]
            tunnel: w336 -> [w355] mode=indexing
            n142 = Number To Fractional String(number=w355, precision (6)=2) -> (F-format string=w354:T13)  [unwired: 2 in]
            n143 = Unbundle By Name(w354) -> ("Rectangle Descriptor.Corners"=w353:cluster{"X":string, "Y":string}[], "Rectangle Descriptor.Angle"=w350:string, "Rectangle Descriptor.Width"=w349:string, "Rectangle Descriptor.Height"=w348:string, "Rectangle Descriptor.Score"=w347:string, "Rectangle Descriptor(Real).Corners"=w345:cluster{"X":string, "Y":string}[], "Rectangle Descriptor(Real).Angle"=w343:string, "Rectangle Descriptor(Real).Width"=w342:string, "Rectangle Descriptor(Real).Height"=w341:string, "Rectangle Descriptor(Real).Score"=w340:string)
            n144 = for {
              N: 4 -> [_]
              tunnel: w353 -> [w366] mode=indexing
              shift-right: [w364] -> w352
              shift-left: string[] [] -> [w363]
              n145 = Cluster To Array(cluster=w366) -> (array=w365:string[])
              n146 = Build Array (concatenate)(w363, w365) -> (w364:string[])
            }
            n147 = for {
              N: 4 -> [_]
              tunnel: w345 -> [w362] mode=indexing
              shift-right: [w360] -> w344
              shift-left: string[] [] -> [w359]
              n148 = Cluster To Array(cluster=w362) -> (array=w361:string[])
              n149 = Build Array (concatenate)(w359, w361) -> (w360:string[])
            }
            n150 = Build Array (concatenate)(w358, w352, w350, w349, w348, w347, w344, w343, w342, w341, w340) -> (w356:string[])
          }
          n151 = Number To Decimal String(number=w333) -> (decimal integer string=w334:string)  [unwired: 1 in]
          n152 = Build Array (concatenate)(w334, w335) -> (w332:string[])
        }
        frame Enabled {
          n153 = for {
            shift-right: [w386] -> w370
            shift-left: w372 -> [w388]
            tunnel: w371 -> [w385] mode=indexing
            n154 = Number To Fractional String(number=w385, precision (6)=2) -> (F-format string=w384:T13)  [unwired: 2 in]
            n155 = Unbundle By Name(w384) -> ("Rectangle Descriptor.Corners"=w383:cluster{"X":string, "Y":string}[], "Rectangle Descriptor.Angle"=w380:string, "Rectangle Descriptor.Width"=w379:string, "Rectangle Descriptor.Height"=w378:string, "Rectangle Descriptor.Score"=w377:string, "Rectangle Descriptor(Real).Corners"=w375:cluster{"X":string, "Y":string}[])  [unwired: 4 out]
            n156 = for {
              N: 4 -> [_]
              tunnel: w383 -> [w396] mode=indexing
              shift-right: [w394] -> w382
              shift-left: string[] [] -> [w393]
              n157 = Cluster To Array(cluster=w396) -> (array=w395:string[])
              n158 = Build Array (concatenate)(w393, w395) -> (w394:string[])
            }
            n159 = for {
              N: 4 -> [_]
              tunnel: w375 -> [w392] mode=indexing
              shift-right: [w390] -> _
              shift-left: string[] [] -> [w389]
              n160 = Cluster To Array(cluster=w392) -> (array=w391:string[])
              n161 = Build Array (concatenate)(w389, w391) -> (w390:string[])
            }
            n162 = Build Array (concatenate)(w388, w382, w380, w379, w378, w377) -> (w386:string[])
          }
          n163 = Number To Decimal String(number=w368) -> (decimal integer string=w369:string)  [unwired: 1 in]
          n164 = Build Array (concatenate)(w369, w370) -> (w367:string[])
        }
      }
    }
    frame "Circles", Default {
      w400 = T14 {"Enum_ShapeType"=enum."Circles", "numbers"=0, "Circle "=[]}  # Circle
      n165 = Variant To Data(type=w400, Variant=w401) -> (data=w397:T14)  [unwired: 1 in, 1 out]
      n166 = Unbundle By Name(w397) -> ("numbers"=w398:i32, "Circle"=w399:T15)
      n167 = disable-structure shown="Enabled" {
        disable-tunnel: string[] [] -> [w406 w483 w498]
        disable-tunnel: [w405 w479 w494] -> w402
        disable-tunnel: w399 -> [_ w481 w496]
        disable-tunnel: w398 -> [_ w480 w495]
        frame Disabled {
          n168 = for {
            N: [_] -> w407
            tunnel: _ -> [w429]
            shift-right: [w431] -> w405
            shift-left: w406 -> [w432]
            tunnel: [w430] -> w404
            i -> [w435]
            w414 = refnum<vi> refnum  # Cluster
            (unwired) dbl[] []
            w419 = refnum<vi> refnum  # Array
            w410 = "_" ("string")
            w445 = refnum<vi> refnum  # Cluster
            n169 = Increment(x=w435) -> (x+1=w434:i32)
            n170 = Number To Decimal String(number=w434) -> (decimal integer string=w428:string)  [unwired: 1 in]
            n171 = property class="Clust (strict)"() -> (reference=w449:refnum<vi>, "Controls[]"=w448:refnum<vi>[])  [unwired: 1 in, 2 out]
            n172 = case shown="True" w430 {
              tunnel: w429 -> [w472 w477]
              tunnel: w428 -> [_ w474]
              tunnel: [w471 w476] -> w411
              tunnel: "PM" ("string") -> [w470 w473]
              frame True {
                n173 = Concatenate Strings(w472, w470, "_" ("string")) -> (w471:string)
              }
              frame False {
                n174 = Concatenate Strings(w477, w473, w474, "_" ("string")) -> (w476:string)
              }
            }
            n175 = Index Array(array=w448) -> (element #1=w447:refnum<vi>, element #2=w426:refnum<vi>, element #3=w425:refnum<vi>, element #4=w438:refnum<vi>, element #5=w418:refnum<vi>)  [unwired: 5 in]
            n176 = To More Specific Class(target class=w445, reference=w447) -> (specific class reference=w446:refnum<vi>)  [unwired: 1 in, 1 out]
            n177 = To More Specific Class(target class=w419, reference=w418) -> (specific class reference=w417:refnum<vi>)  [unwired: 1 in, 1 out]
            n178 = property class="Arr"(reference=w417) -> ("Label.Text"=w416:string, "Array Element"=w413:refnum<vi>)  [unwired: 1 in, 2 out]
            n179 = property class="Clust"(reference=w446) -> ("Label.Text"=w441:string, "Controls[]"=w444:refnum<vi>[])  [unwired: 1 in, 2 out]
            n180 = property class="Ctl"(reference=w426) -> ("Label.Text"=w424:string)  [unwired: 1 in, 2 out]
            n181 = property class="Ctl"(reference=w425) -> ("Label.Text"=w423:string)  [unwired: 1 in, 2 out]
            n182 = property class="Ctl"(reference=w438) -> ("Label.Text"=w433:string)  [unwired: 1 in, 2 out]
            n183 = To More Specific Class(target class=w414, reference=w413) -> (specific class reference=w412:refnum<vi>)  [unwired: 1 in, 1 out]
            n184 = Index Array(array=w444) -> (element #1=w443:refnum<vi>, element #2=w442:refnum<vi>)  [unwired: 2 in]
            n185 = for {
              N: 4 -> [_]
              tunnel: w416 -> [w454]
              tunnel: w412 -> [w468]
              tunnel: w411 -> [w461]
              tunnel: w410 -> [w460]
              shift-right: [w456] -> w408
              shift-left: string[] [] -> [w459]
              i -> [w455]
              w467 = "_" ("string")
              n186 = property class="Clust"(reference=w468) -> ("Controls[]"=w462:refnum<vi>[])  [unwired: 1 in, 2 out]
              n187 = Number To Decimal String(number=w455) -> (decimal integer string=w452:string)  [unwired: 1 in]
              n188 = Index Array(array=w462) -> (element #1=w463:refnum<vi>, element #2=w464:refnum<vi>)  [unwired: 2 in]
              n189 = property class="Ctl"(reference=w463) -> ("Label.Text"=w465:string)  [unwired: 1 in, 2 out]
              n190 = property class="Ctl"(reference=w464) -> ("Label.Text"=w466:string)  [unwired: 1 in, 2 out]
              n191 = Concatenate Strings(w454, "[" ("string"), w452, "]" ("string")) -> (w450:string)
              n192 = Concatenate Strings(w461, w460, w450, w467, w465) -> (w458:string)
              n193 = Concatenate Strings(w461, w460, w450, w467, w466) -> (w457:string)
              n194 = Build Array (concatenate)(w459, w458, w457) -> (w456:string[])
            }
            n195 = property class="Ctl"(reference=w443) -> ("Label.Text"=w440:string)  [unwired: 1 in, 2 out]
            n196 = property class="Ctl"(reference=w442) -> ("Label.Text"=w439:string)  [unwired: 1 in, 2 out]
            n197 = Concatenate Strings(w411, w441, w410, w440) -> (w437:string)
            n198 = Concatenate Strings(w411, w441, w410, w439) -> (w436:string)
            n199 = Concatenate Strings(w411, w424) -> (w420:string)
            n200 = Concatenate Strings(w411, w423) -> (w421:string)
            n201 = Concatenate Strings(w411, w433) -> (w422:string)
            n202 = Build Array (concatenate)(w432, w437, w436, w420, w421, w422, w408) -> (w431:string[])
          }
        }
        frame Enabled {
          n203 = for {
            shift-right: [w484] -> w482
            shift-left: w483 -> [w492]
            tunnel: w481 -> [w490] mode=indexing
            n204 = Number To Fractional String(number=w490, precision (6)=2) -> (F-format string=w489:T16)  [unwired: 2 in]
            n205 = Unbundle By Name(w489) -> ("Circle Descriptor.Position.X"=w488:string, "Circle Descriptor.Position.Y"=w487:string, "Circle Descriptor.Radius"=w486:string, "Circle Descriptor.Score"=w485:string)  [unwired: 4 out]
            n206 = Build Array (concatenate)(w492, w488, w487, w486, w485) -> (w484:string[])
          }
          n207 = Number To Decimal String(number=w480) -> (decimal integer string=w478:string)  [unwired: 1 in]
          n208 = Build Array (concatenate)(w478, w482) -> (w479:string[])
        }
        frame Disabled {
          n209 = for {
            shift-right: [w499] -> w497
            shift-left: w498 -> [w511]
            tunnel: w496 -> [w509] mode=indexing
            n210 = Number To Fractional String(number=w509, precision (6)=2) -> (F-format string=w508:T16)  [unwired: 2 in]
            n211 = Unbundle By Name(w508) -> ("Circle Descriptor.Position.X"=w507:string, "Circle Descriptor.Position.Y"=w506:string, "Circle Descriptor.Radius"=w505:string, "Circle Descriptor.Score"=w504:string, "Circle Descriptor(Real).Position.X"=w503:string, "Circle Descriptor(Real).Position.Y"=w502:string, "Circle Descriptor(Real).Radius"=w501:string, "Circle Descriptor(Real).Score"=w500:string)
            n212 = Build Array (concatenate)(w511, w507, w506, w505, w504, w503, w502, w501, w500) -> (w499:string[])
          }
          n213 = Number To Decimal String(number=w495) -> (decimal integer string=w493:string)  [unwired: 1 in]
          n214 = Build Array (concatenate)(w493, w497) -> (w494:string[])
        }
      }
    }
  }
  "ResultValues" <- w4
